vi "Is Empty.vi"(8 "error in (no error)":errorcluster, 11 "Abs_Waveform in":refnum<class "Abs_Waveform.lvclass">) -> (0 "error out":errorcluster, 2 "Empty?":bool, 3 "Abs_Waveform out":refnum<class "Abs_Waveform.lvclass">)   [LabVIEW 2021, in "Abs_Waveform.lvclass"]
uses:
  Abs_Waveform.lvclass
  Abs_Waveform.lvclass/Abs_Waveform.ctl
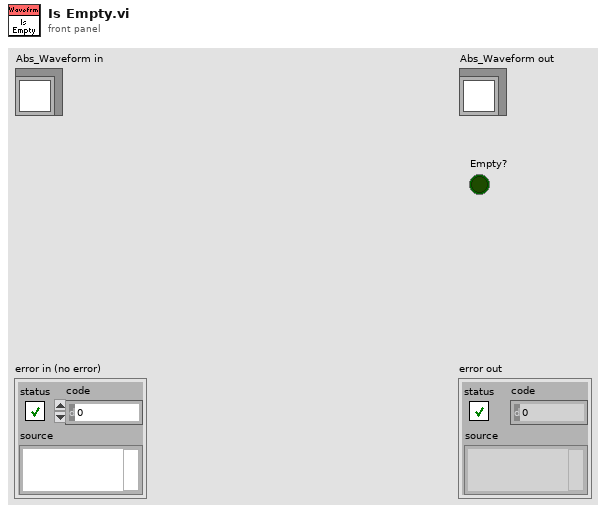
[diagram p1: front panel]
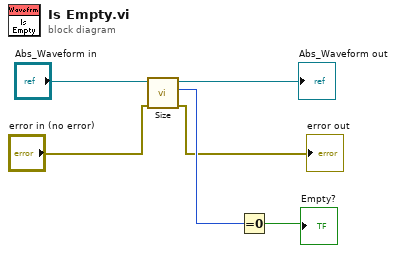
[diagram p0: block diagram]
diagram:
  n1 = call-dynamic "Size.vi"("error in (no error)"="error in (no error)", "Abs_Waveform in"="Abs_Waveform in") -> ("error out"=→"error out":errorcluster, "size"=w3:i32, "Abs_Waveform out"=→"Abs_Waveform out":refnum<class "Abs_Waveform.lvclass">)  [unwired: 7 in]
  n2 = Equal To 0?(x=w3) -> (x = 0?=→"Empty?":bool)
